vi "select scaled data.vi"(10 "Sensor index":u32, 11 "Sensor Data":T1 {"Sensor array"."scaled" format="%.2f"; "Sensor array"."voltage" format="%.4f"; "Time" format="%<%I:%M:%S%2u %p\n%m/%d/%Y>T"}) -> (1 "voltage":sgl format="%.5f", 2 "units":string, 3 "scaled":sgl format="%.2f", 4 "Time":dbl format="%.2f", 5 "number of sensors":i32, 6 "Out of Range":bool)   [LabVIEW 2015]
doc: "Unbundles the Sensor data cluster based on the selected sensor and outputs the scaled data, units, out of range error, and arbitrary time from the Data server."
uses:
  TCP DAQ/Sensor data.ctl
  sensor cluster.ctl
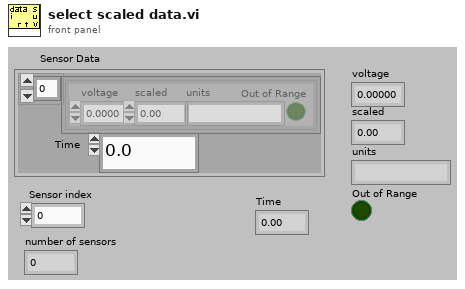
[diagram p1: front panel]
types:
  T1 = typedef "Sensor data.ctl" = cluster{" Sensor array":T2[], "Time":dbl}
  T2 = typedef "sensor cluster.ctl" = cluster{"voltage":sgl, "scaled":sgl, "units":string, "Out of Range":bool}
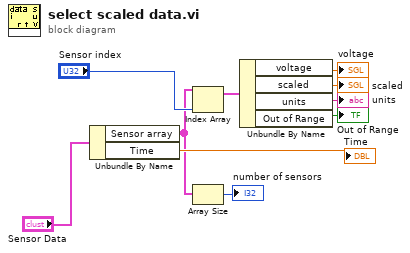
[diagram p0: block diagram]
diagram:
  n1 = Unbundle By Name("Sensor Data") -> ("Sensor array"=w2:T2[], "Time"=→"Time":dbl)
  n2 = Index Array(array=w2, index="Sensor index") -> (element=w7:T2)
  n3 = Array Size(array=w2) -> (size(s)=→"number of sensors":i32)
  n4 = Unbundle By Name(w7) -> ("voltage"=→"voltage":sgl, "scaled"=→"scaled":sgl, "units"=→"units":string, "Out of Range"=→"Out of Range":bool)
